vi "ATS9350_NPT.vi"() -> ()   [LabVIEW 2018]
panel:
  out "Graph":u16[](graph)
  in  "stop":bool
  # "Connect proper signal to channel A before starting acquisition\n(e.g. 1Vpp 1kHz sine wave)"
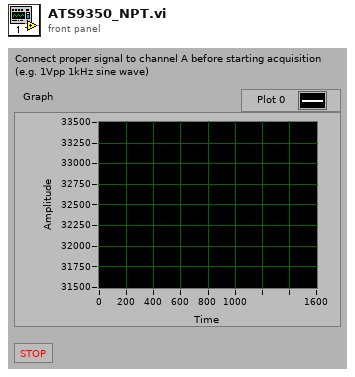
[diagram p1: front panel]
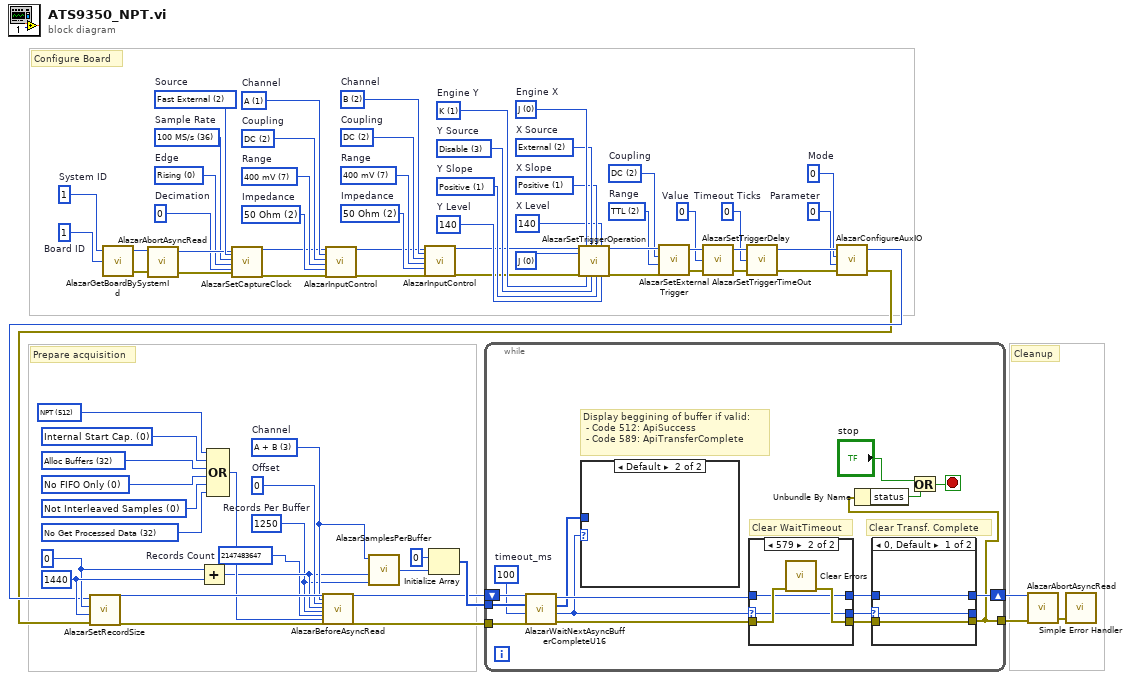
[diagram p0: block diagram]
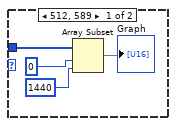
[diagram p2: hidden frame]
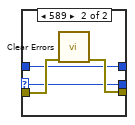
[diagram p3: hidden frame]
diagram:
  w1 = u32 2147483647  # Records Count
  w36 = u32 2 items=["50 Ohm"=2]  # Impedance
  w35 = u32 7 items=["40 mV"=2, "100 mV"=5, "200 mV"=6, "400 mV"=7, "1 V"=10, "2 V"=11, "4 V"=12]  # Range
  w37 = u32 2 items=["AC"=1, "DC"=2]  # Coupling
  w38 = u8 2 items=["A"=1, "B"=2, "C"=4, "D"=8]  # Channel
  w14 = u32 0  # Parameter
  w13 = u32 0  # Mode
  w12 = u32 0  # Timeout Ticks
  w19 = u32 0  # Value
  w23 = u32 2 items=["5 V", "1 V", "TTL"]  # Range
  w22 = u32 2 items=["AC"=1, "DC"=2]  # Coupling
  w26 = u32 140  # Y Level
  w27 = u32 1 items=["Positive"=1, "Negative"=2]  # Y Slope
  w28 = u32 3 items=["A", "B", "External", "Disable", "C", "D"]  # Y Source
  w30 = u32 140  # X Level
  w31 = u32 1 items=["Positive"=1, "Negative"=2]  # X Slope
  w32 = u32 2 items=["A", "B", "External", "Disable", "C", "D"]  # X Source
  w29 = u32 1 items=["J", "K"]  # Engine Y
  w33 = u32 0 items=["J", "K"]  # Engine X
  w34 = u32 0 items=["J", "K", "J OR K", "J AND K", "J XOR K", "J AND NOT K", "NOT J AND K"] ("Op.")
  w41 = u32 2 items=["50 Ohm"=2]  # Impedance
  w42 = u32 7 items=["40 mV"=2, "100 mV"=5, "200 mV"=6, "400 mV"=7, "1 V"=10, "2 V"=11, "4 V"=12]  # Range
  w43 = u32 2 items=["AC"=1, "DC"=2]  # Coupling
  w44 = u8 1 items=["A"=1, "B"=2, "C"=4, "D"=8]  # Channel
  w46 = u32 0  # Decimation
  w47 = u32 0 items=["Rising", "Falling"]  # Edge
  w48 = u32 36 items=["1 kS/s"=1, "2 kS/s"=2, "5 kS/s"=4, "10 kS/s"=8, "20 kS/s"=10, "50 kS/s"=12, "100 kS/s"=14, "200 kS/s"=16, "500 kS/s"=18, "1 MS/s"=20, "2 MS/s"=24, "5 MS/s"=26, "10 MS/s"=28, "20 MS/s"=30, "50 MS/s"=34, "100 MS/s"=36, "125 MS/s"=37, "250 MS/s"=43, "500 MS/s"=48, "USER_DEF"=0]  # Sample Rate
  w50 = u32 2 items=["Internal"=1, "Fast External"=2, "Medium External"=3, "Slow External"=4, "External AC"=5, "External DC"=6, "External 10MHz"=7]  # Source
  w54 = u32 1  # Board ID
  w53 = u32 1  # System ID
  w2 = u32 1250  # Records Per Buffer
  w62 = u32 0  # Offset
  w4 = u32 3 items=["A"=1, "B"=2, "A + B"=3, "C"=4, "A + C"=5, "A + B"=6, "D"=8, "A + D"=9, "B + D"=10, "C + D"=12, "A + B + C + D"=15]  # Channel
  w67 = u32 1440 ("Post-trigger Samples")
  w66 = u32 0 ("Pre-trigger Samples")
  w73 = u32 32 items=["No Get Processed Data"=32, "Get Processed Data"=8192]
  w72 = u32 0 items=["Not Interleaved Samples"=0, "Interleave Samples"=4096]
  w68 = u32 0 items=["No FIFO Only"=0, "FIFO Only"=2048]
  w71 = u32 32 items=["Alloc Buffers"=32]
  w70 = u32 0 items=["Internal Start Cap.", "External Start Cap."]
  w69 = u32 512 items=["Traditional"=0, "NPT"=512, "Continuous"=256, "Triggered Streaming"=1024]
  # "Configure Board"
  # "Cleanup"
  # "Prepare acquisition"
  n1 = call "AlazarGetBoardBySystemId.vi"("Board ID"=w54, "System ID"=w53) -> ("error out"=w51:errorcluster, "Handle"=w52:u64)  [unwired: 1 in, 1 out]
  n2 = call "AlazarAbortAsyncRead.vi"("Handle"=w52, "error in (no error)"=w51) -> ("Handle"=w49:u64, "error out"=w45:errorcluster)  [unwired: 1 out]
  n3 = Add(x=w66, y=w67) -> (x+y=w3:u32)
  n4 = Compound Arithmetic op=OR(w69, w70, w71, w68, w72, w73) -> (w63:u32)
  n5 = call "AlazarSetCaptureClock.vi"("Handle"=w49, "Source"=w50, "Sample Rate"=w48, "Edge"=w47, "Decimation"=w46, "error in (no error)"=w45) -> ("Handle"=w40:u64, "error out"=w39:errorcluster)  [unwired: 11 in, 1 out]
  n6 = call "AlazarInputControl.vi"("Handle"=w40, "Channel"=w44, "Coupling"=w43, "Range"=w42, "Impedance"=w41, "error in (no error)"=w39) -> ("Handle"=w11:u64, "error out"=w10:errorcluster)  [unwired: 11 in, 1 out]
  n7 = call "AlazarSamplesPerBuffer.vi"("Records Per Buffer"=w2, "Samples Per Record"=w3, "Channel Mask"=w4) -> ("Samples Per Buffer"=w5:u32)  [unwired: 1 in]
  n8 = call "AlazarInputControl.vi"("Handle"=w11, "Channel"=w38, "Coupling"=w37, "Range"=w35, "Impedance"=w36, "error in (no error)"=w10) -> ("Handle"=w8:u64, "error out"=w9:errorcluster)  [unwired: 11 in, 1 out]
  n9 = Initialize Array(u16 0, w5) -> (w60:u16[])
  n10 = call "AlazarSetTriggerOperation.vi"("Handle"=w8, "Trigger Operation"=w34, "error in (no error)"=w9, "Trigger Engine 1"=w33, "Trigger Engine 2"=w29, "Source 1"=w32, "Source 2"=w28, "Slope 1"=w31, "Slope 2"=w27, "Level 1"=w30, "Level 2"=w26) -> ("Handle"=w25:u64, "error out"=w24:errorcluster)  [unwired: 6 in, 1 out]
  n11 = call "AlazarSetExternalTrigger.vi"("error in (no error)"=w24, "Range ID"=w23, "Coupling ID"=w22, "Handle"=w25) -> ("error out"=w20:errorcluster, "Handle"=w21:u64)  [unwired: 1 out]
  n12 = call "AlazarSetTriggerDelay.vi"("error in (no error)"=w20, "Delay"=w19, "Handle"=w21) -> ("error out"=w17:errorcluster, "Handle"=w18:u64)  [unwired: 1 out]
  n13 = call "AlazarSetTriggerTimeOut.vi"("error in (no error)"=w17, "Timeout Ticks"=w12, "Handle"=w18) -> ("error out"=w15:errorcluster, "Handle"=w16:u64)  [unwired: 1 out]
  n14 = call "AlazarConfigureAuxIO.vi"("error in (no error)"=w15, "Parameter"=w14, "Mode"=w13, "Handle"=w16) -> ("error out"=w6:errorcluster, "Handle"=w7:u64)  [unwired: 1 out]
  n15 = call "AlazarSetRecordSize.vi"("error in (no error)"=w6, "Post-trigger Samples"=w67, "Pre-trigger Samples"=w66, "Handle"=w7) -> ("error out"=w64:errorcluster, "Handle"=w65:u64)  [unwired: 1 out]
  n16 = call "AlazarBeforeAsyncRead.vi"("Handle"=w65, "Channel Select"=w4, "Transfer Offset"=w62, "Transfer Length"=w3, "Records Per Buffer"=w2, "Records Per Acquisition"=w1, "Flags"=w63, "error in (no error)"=w64) -> ("Handle"=w59:u64, "error out"=w58:errorcluster)  [unwired: 17 in, 1 out]
  n17 = while {
    tunnel: w60 -> [w89]
    tunnel: w58 -> [w86]
    tunnel: [w74] -> w55
    shift-right: [w79] -> w56
    shift-left: w59 -> [w88]
    stop <- w82 stop-if-true
    w87 = u32 100  # timeout_ms
    # "Display beggining of buffer if valid:\n - Code 512: ApiSuccess\n - Code 589: ApiTransferComplete"
    # "Clear Transf. Complete"
    # "Clear WaitTimeout"
    n18 = call "AlazarWaitNextAsyncBufferCompleteU16.vi"("error in (no error)"=w86, "Timeout (ms)"=w87, "Buffer"=w89, "Handle"=w88) -> ("error out"=w76:errorcluster, "Return Code"=w75:u32, "Buffer"=w77:u16[], "Handle"=w78:u64)
    n19 = case shown="Default" w75 {
      tunnel: w77 -> [w90 _]
      frame 512, 589 {
        n20 = Array Subset(array=w90, index=0, length=1440) -> (→"Graph":u16[])
      }
      frame Default {
      }
    }
    n21 = case shown="579" w75 {
      selector: w75 -> [w102 w104]
      tunnel: w76 -> [w101 w107]
      tunnel: [w101 w106] -> w85
      tunnel: [w103 w105] -> w84
      tunnel: w78 -> [w103 w105]
      tunnel: [w102 w104] -> w83
      frame 0, Default {
      }
      frame 579 {
        n22 = call <vilib>:"Clear Errors.vi"("error in (no error)"=w107) -> ("error out"=w106:errorcluster)  [unwired: 5 in, 1 out]
      }
    }
    n23 = case shown="0, Default" w83 {
      selector: w83 -> [w95 w97]
      tunnel: w85 -> [w94 w100]
      tunnel: [w94 w99] -> w74
      tunnel: [w96 w98] -> w79
      tunnel: w84 -> [w96 w98]
      tunnel: [w95 w97] -> _
      frame 0, Default {
      }
      frame 589 {
        n24 = call <vilib>:"Clear Errors.vi"("error in (no error)"=w100) -> ("error out"=w99:errorcluster)  [unwired: 5 in, 1 out]
      }
    }
    n25 = Unbundle By Name(w74) -> ("status"=w80:bool)
    n26 = Or(x="stop", y=w80) -> (x .or. y?=w82:bool)
  }
  n27 = call "AlazarAbortAsyncRead.vi"("Handle"=w56, "error in (no error)"=w55) -> ("error out"=w57:errorcluster)  [unwired: 2 out]
  n28 = call <vilib>:"Simple Error Handler.vi"("error in (no error)"=w57) -> ()  [unwired: 4 in, 5 out]
